vi "BlinkingLED_Main.vi"() -> ()   [LabVIEW 2014]
uses:
  <vilib>/MakerHub/LINX/Public/Peripherals/Digital/Digital Write 1 Chan.vi
  <vilib>/MakerHub/LINX/Public/Peripherals/Digital/Digital Write N Chans.vi
  <vilib>/MakerHub/LINX/Private/Local IO/LinxDigitalWrite.vi
  <vilib>/MakerHub/LINX/Public/Utilities/Check Channel.vi
  <vilib>/MakerHub/LINX/Private/Local IO/Handle Errors.vi
  <vilib>/MakerHub/LINX/Public/Utilities/Open Local.vi
  <vilib>/MakerHub/LINX/Private/Utilties/Generate Error.vi
  <vilib>/MakerHub/LINX/LMH-LINX.lvlib
panel:
  out "Error Out":errorcluster
  out "LED":bool
  in  "Stop":bool
  # "Blinking LED on Pin 7 (GPIO 4)"
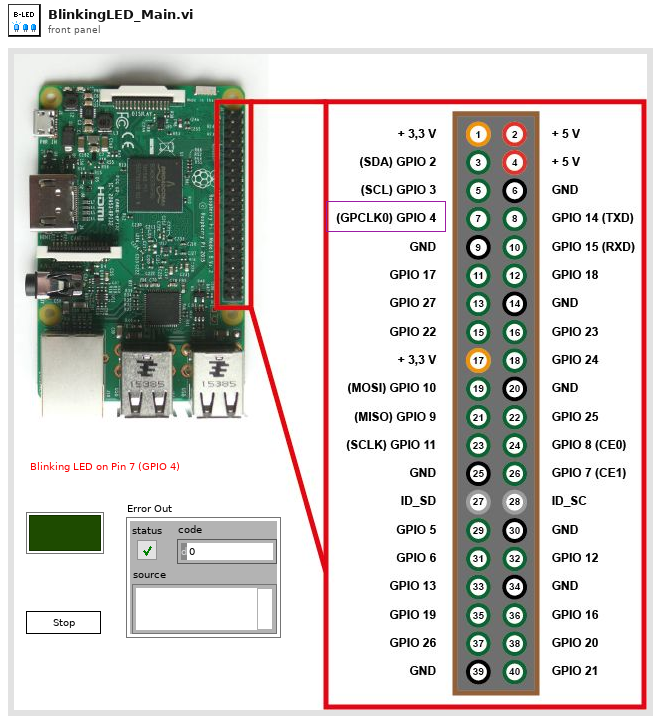
[diagram p1: front panel]
types:
  T1 = typedef "LMH-LINX.lvlib/LINX Ref.ctl" = cluster{"IO":T2, "Interface":T3, "LINX Device Config":T4}
  T2 = typedef "LMH-LINX.lvlib/Platform.ctl" = enum16{"Remote", "Local"}
  T3 = typedef "LMH-LINX.lvlib/Interface.ctl" = enum16{"Serial", "TCP"}
  T4 = typedef "LMH-LINX.lvlib/Device.lvlib/LINX Device Config.ctl" = cluster{"Interface":T3, "COM Port":refnum<visa-resource-name>, "TCP Configuration":T5, "Device Family":u8, "Device ID":u8, "Device Name":string, "TCP Ref":refnum<k5>, "Channels":T6}
  T5 = typedef "LMH-LINX.lvlib/Device.lvlib/TCP Config.ctl" = cluster{"IP Address":string, "Port":u16}
  T6 = typedef "LMH-LINX.lvlib/Channels.ctl" = cluster{"DI":u8[], "DO":u8[], "AI":u8[], "AO":u8[], "PWM":u8[], "QE":u8[], "UART":u8[], "I2C 2":u8[], "SPI":u8[], "CAN":u8[], "Servo":u8[], "AI Ref (V)":dbl, "AI Resolution (Bits)":u8, "AO Ref (V)":dbl, "AO Resolution (Bits)":u8}
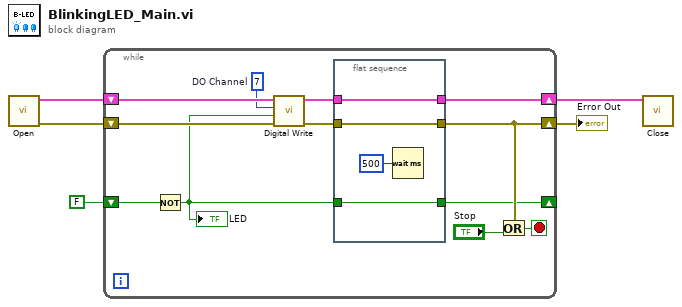
[diagram p0: block diagram]
diagram:
  n1 = call-poly <vilib>:"Open.vi"() -> ("Error Out"=w5:errorcluster, "LINX Resource"=w4:T1)  [unwired: 9 in, 1 out]
  n2 = while {
    shift-right: [w7] -> w2
    shift-left: w4 -> [w9]
    shift-right: [w14] -> w1
    shift-left: w5 -> [w12]
    shift-right: [w13] -> _
    shift-left: FALSE -> [w15]
    stop <- w16 stop-if-true
    w6 = u8 7  # DO Channel
    n3 = Not(x=w15) -> (.not. x?=w10:bool)
    "LED" <- w10
    n4 = call-poly <vilib>:"Digital Write.vi"("Error In"=w12, "Output Value"=w10, "DO Channel"=w6, "LINX Resource"=w9) -> ("Error Out"=w11:errorcluster, "LINX Resource"=w8:T1)  [unwired: 6 in]
    n5 = flat-sequence {
      tunnel: [w18] -> w14
      tunnel: w11 -> [w18]
      tunnel: w10 -> [w21]
      tunnel: [w21] -> w13
      tunnel: w8 -> [w19]
      tunnel: [w19] -> w7
      frame #0 {
        n6 = Wait (ms)(milliseconds to wait=u32 500) -> ()  [unwired: 1 out]
      }
    }
    n7 = Or(x=w14, y="Stop") -> (x .or. y?=w16:bool)
  }
  "Error Out" <- w1
  n8 = call <vilib>:"Close.vi"("LINX Resource"=w2) -> ()  [unwired: 10 in, 1 out]
